vi "VerifyIEPaths.vi"() -> ()   [LabVIEW 2021]
uses:
  <vilib>/Wiresmith Technology/G CLI/CLI Class/CLI.lvclass
panel:
  out "error out":errorcluster
  in  "Manual Test":bool
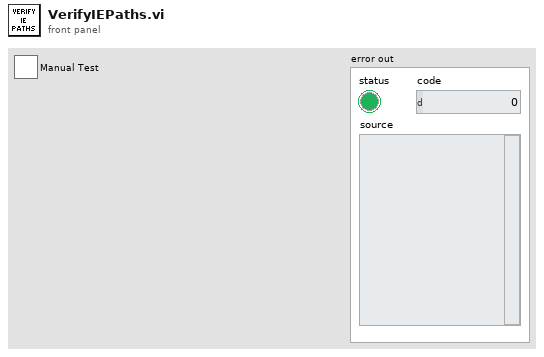
[diagram p1: front panel]
types:
  T1 = enum16{"open", "replace", "create", "open or create", "replace or create", "replace or create with confirmation"}
  T2 = enum32{"Invalid", "Standard", "Closed", "Hidden", "Minimized", "Maximized"}
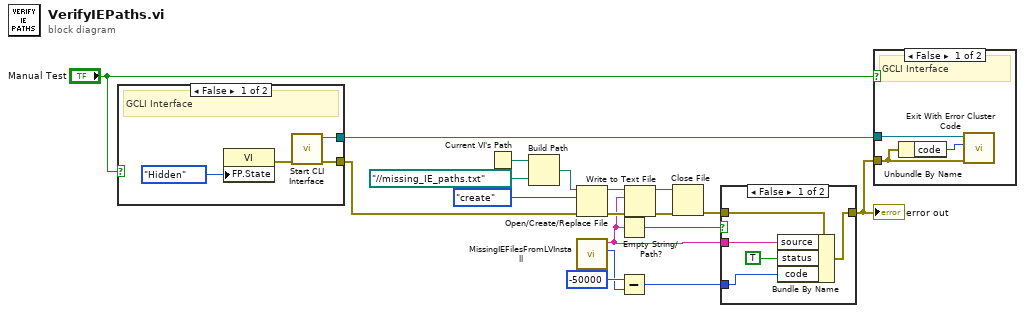
[diagram p0: block diagram]
diagram:
  n1 = case shown="False" "Manual Test" {
    tunnel: [w21 _] -> w15
    tunnel: [w19 _] -> w1
    frame False {
      # "GCLI Interface"
      n2 = property class="VI"("FP.State"=T2."Hidden" ("Front Panel Window:State")) -> (error out=w22:errorcluster)  [unwired: 2 in, 1 out]
      n3 = call <vilib>:"Start CLI Interface.vi"("error in (no error)"=w22) -> ("error out"=w21:errorcluster, "CLI out"=w19:refnum<class "CLI.lvclass">)  [unwired: 7 in, 2 out]
    }
    frame True {
      # "Running Manual"
    }
  }
  n4 = Current VI's Path() -> (path=w3:path)
  n5 = Build Path(base path=w3, name or relative path=path "../../missing_IE_paths.txt") -> (appended path=w11:path)
  n6 = Open/Create/Replace File(file path (use dialog)=w11, error in=w15, operation (0:open)=T1."create") -> (refnum out=w8:refnum<file>, error out=w18:errorcluster)  [unwired: 3 in, 1 out]
  n7 = call "MissingIEFilesFromLVInstall.vi"() -> ("Code"=w5:i32, "Missing IE Paths"=w7:string)  [unwired: 10 in]
  n8 = Empty String/Path?(string/path=w7) -> (empty?=w9:bool)
  n9 = Subtract(x=-50000 ("code"), y=w5) -> (x-y=w4:i32)
  n10 = Write to Text File(file (use dialog)=w8, text=w7, error in=w18) -> (refnum out=w13:refnum<file>, error out=w17:errorcluster)  [unwired: 1 in, 1 out]
  n11 = Close File(refnum=w13, error in=w17) -> (error out=w16:errorcluster)  [unwired: 1 out]
  n12 = case shown="False" w9 {
    tunnel: w16 -> [w27 w28]
    tunnel: w7 -> [w24 _]
    tunnel: [w26 w28] -> w14
    tunnel: w4 -> [w23 _]
    frame False {
      n13 = Bundle By Name(cluster=w27, "source"=w24, "status"=TRUE, "code"=w23) -> (w26:errorcluster)
    }
    frame True {
    }
  }
  "error out" <- w14
  n14 = case shown="False" "Manual Test" {
    tunnel: w1 -> [w30 _]
    tunnel: w14 -> [w31 _]
    frame False {
      # "GCLI Interface"
      n15 = Unbundle By Name(w31) -> ("code"=w29:i32)
      n16 = call <vilib>:"Exit With Error Cluster Code.vi"("error in (no error)"=w31, "No Error Code (0)"=w29, "CLI in"=w30) -> ()  [unwired: 8 in, 1 out]
    }
    frame True {
      # "Running Manual"
    }
  }
